vi "TPM with correction version 10-3-compare-1 scale factor_descan_20191023_WF.vi"() -> ()   [LabVIEW 2018]
uses:
  Casao LabVIEW SDK 1.0.5/Haso/Data Haso/Wavefront parameters.ctl
  Casao LabVIEW SDK 1.0.5/Casao/Casao/Loop prefs.ctl
  Casao LabVIEW SDK 1.0.5/Haso/Data Haso/DataHaso.ctl
  <vilib>/Utility/file.llb/Read From Spreadsheet File (DBL).vi
  <vilib>/Utility/file.llb/Write To Spreadsheet File (DBL).vi
panel:
  in  "galvo scan?":bool
  out "error out 1":errorcluster={"status"=FALSE, "code"=25, "source"=""}
  out "error out 3":errorcluster={"status"=FALSE, "code"=25, "source"=""}
  out "error out 2":errorcluster={"status"=FALSE, "code"=25, "source"=""}
  out "error out 0":errorcluster={"status"=FALSE, "code"=25, "source"=""}
  in  "Descan  Rescan":bool
  in  "Camera              WF sensor":bool
  in  "Scale factor":dbl=1.0
  out "output path":path
  out "Model Coefficients (µm) after":sgl[](array[numeric])
  out "Model Coefficients (µm) before":sgl[](array[numeric])
  in  "stop":bool
  out "Slice now":dbl
  in  "Iteration #":u16(ring)=1 items=["1"=1, "2"=2, "3"=3, "4"=4, "5"=5]
  in  "AoExp Time":dbl(ring)=0.5 items=["0.2s"=0.2, "0.5s"=0.5, "1.0s"=1.0, "1.5s"=1.5]
  out "after correction":T1
  in  "Filter y tilt":bool=TRUE
  in  "Filter x tilt":bool=TRUE
  in  "Curvature filter":bool=TRUE
  out "PV":dbl
  out "RMS":dbl
  in  "Matrix path":path=path "C:/Users/user/Desktop/YD/20191025/CM.aomc"
  in  "Offset path":path=path "D:/SystemAlignment/syste_aberration_20191015.dat"
  out "Camera image":u32[][](graph)
  out "RMS":dbl
  out "PV":dbl
  out "before correction":T1
  in  "Curvature filter":bool=TRUE
  in  "Filter y tilt":bool=TRUE
  in  "Filter x tilt":bool=TRUE
  out "after correction":dbl[][](graph) caption="Wavefront"
  out "before correction":dbl[][](graph) caption="Wavefront"
  in  "ImExp Time (s)":dbl(ring)=0.5 items=["0.2"=0.2, "0.5"=0.5, "1.0"=1.0, "4.0"=4.0, "8.0"=8.0]
  in  "Step size(um)":dbl
  in  "Laser Power%(0-100)":dbl=50.0
  in  "Slices #":dbl=1.0
  in  "Average Frame #":dbl=5.0
  in  "Correction":bool
  # "OFF"
  # "ON"
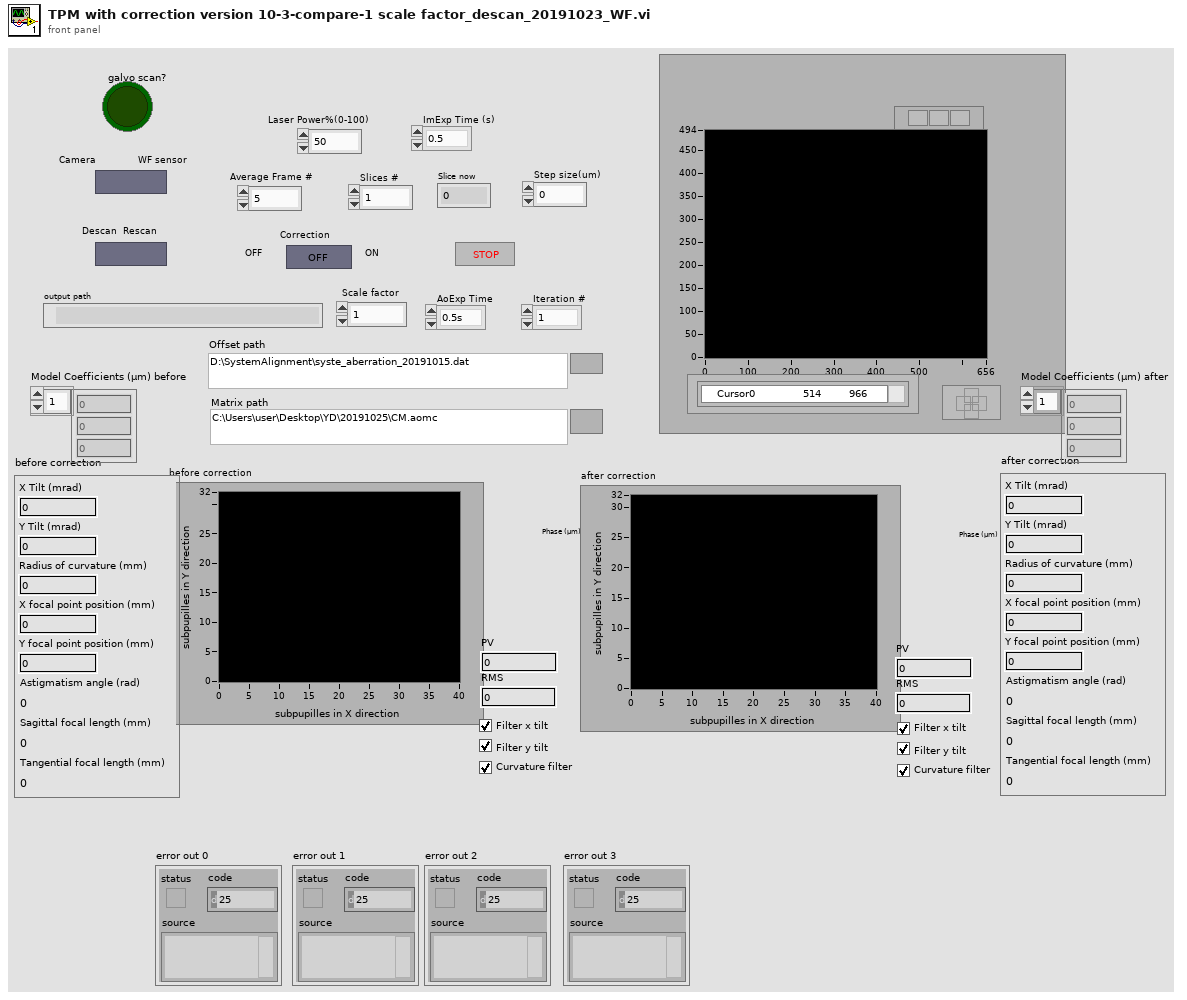
[diagram p1: front panel]
types:
  T1 = typedef "Wavefront parameters.ctl" = cluster{"X Tilt (mrad)":sgl, "Y Tilt (mrad)":sgl, "Radius of curvature (mm)":sgl, "X focal point position (mm)":sgl, "Y focal point position (mm)":sgl, "Astigmatism angle (rad)":sgl, "Sagittal focal length (mm)":sgl, "Tangential focal length (mm)":sgl}
  T2 = typedef "Loop prefs.ctl" = cluster{"Filter tilt on measurement (closed loop)":bool, "Correction gain (closed loop)":sgl, "Limit of subapertures off in CGP (%)":sgl, "Limit of saturated actuators (%)":sgl}
  T3 = cluster{"Filtre tilt X":bool, "Filtre tilt Y":bool, "Filtre courbure":bool}
  T4 = typedef "DataHaso.ctl" = i32
  T5 = cluster{"Measurement":T4, "Target":T4, "Manual target":T4}
  T6 = cluster{"Target for tilt":T4, "Target for focus":T4, "Target for all other aberrations":T4}
  T7 = typedef "Camera.ctl" = i32
  T8 = typedef "PhaseModul.ctl" = i32
  T9 = typedef "Haso.ctl" = i32
  T10 = typedef "Casao.ctl" = i32
  T11 = typedef "Image Compat.ctl" = cluster{"Signed/unsigned":bool, "Number of bits":T12, "Internal object id":i32, "Internal data id":i32}
  T12 = typedef "Data alignment enum.ctl" = enum16{"8", "16", "32"}
  T13 = typedef "Reconstruction prefs.ctl" = cluster{"Reconstruction type":enum16{"Modal", "Zonal"}, "Polynomial type":enum16{"Zernike", "Legendre"}, "Modal reconstruction prefs":T14, "Zonal reconstruction prefs":T17}
  T14 = typedef "Modal reconstruction prefs.ctl" = cluster{"Number of coefficients":u32, "Filtered coefficients":u32[], "RMS Zernike normalization":bool, "Matrix inversion method":u16, "Add zonal residual to modal fit ":bool, "Detection prefs":T15}
  T15 = typedef "PupilDetectionPrefs.ctl" = cluster{"Automatic pupil detection":bool, "Central occultation pupil":bool, "Semi-automatic pupil detection (find radius)":bool, "Semi-automatic pupil detection (find center)":bool, "Automatic pupil detection mode":enum16{"Contained", "Containing"}, "Start coordinates":cluster{"Pupil center (Zernike)":T16, "Pupil radius (Zernike)":sgl, "Pupil center (Legendre)":T16, "Pupil halfsize (Legendre)":T16}}
  T16 = typedef "Point2Df.ctl" = cluster{"X":sgl, "Y":sgl}
  T17 = typedef "Zonal reconstruction prefs.ctl" = cluster{"Number of weak iterations":u16, "Number of max iterations":u32, "Residual limit":sgl}
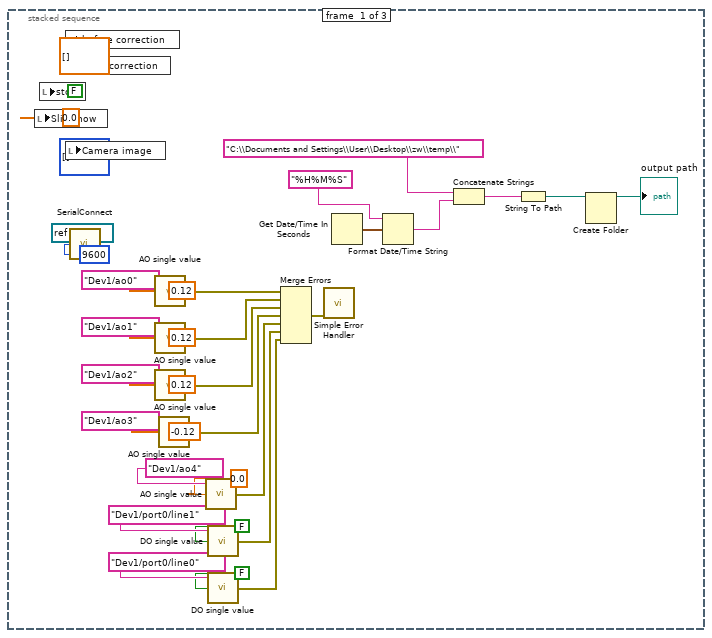
[diagram p2: hidden frame]
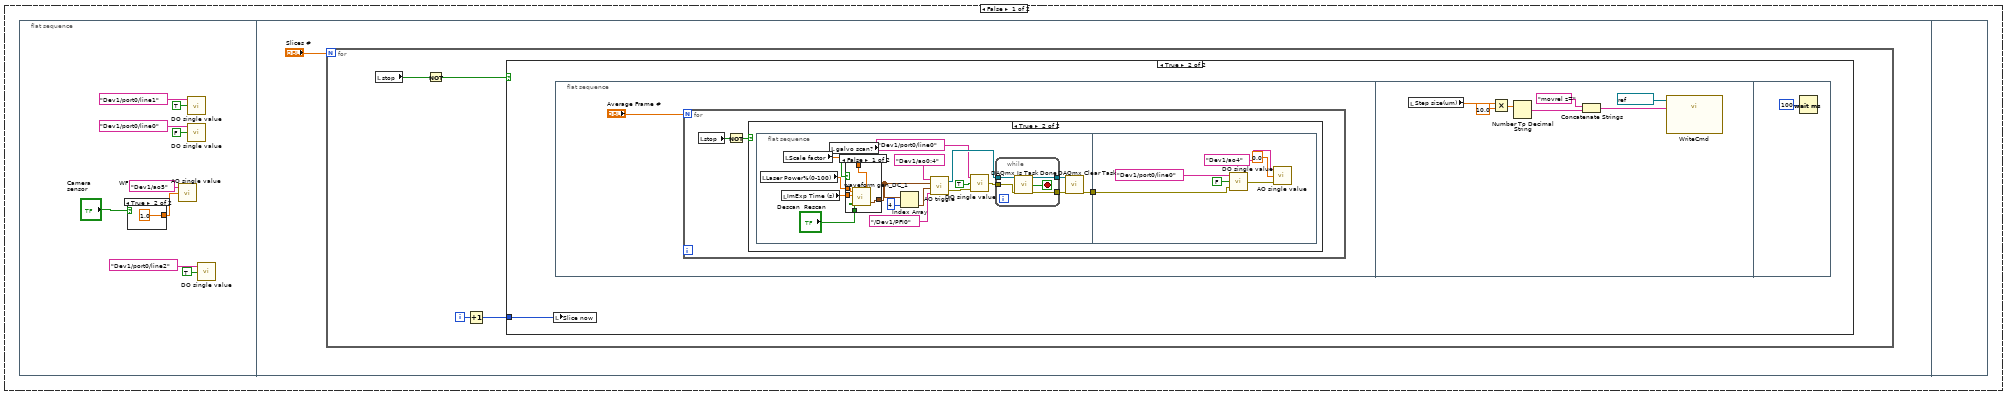
[diagram p3: hidden frame]
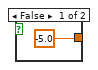
[diagram p4: hidden frame]
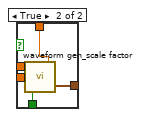
[diagram p7: hidden frame]
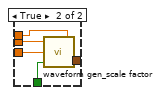
[diagram p10: hidden frame]
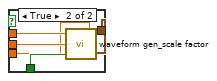
[diagram p11: hidden frame]
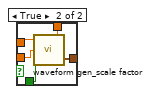
[diagram p12: hidden frame]
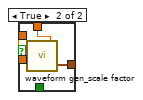
[diagram p16: hidden frame]
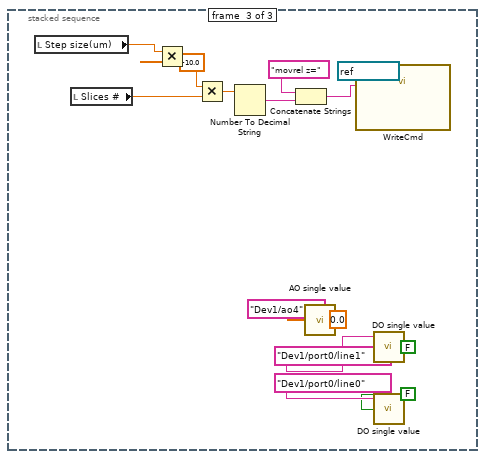
[diagram p17: hidden frame]
diagram:
  # "ao0: stim G A \nao1: stim G B\nao2: Emission G A\nao3: Emission G B\nao4: Pockel Cell\nao5: Emission steering G\nao6: stage z piezo\nPFI0: andor send out trigger\nP0.0: andor send in trigger?"
  n1 = stacked-sequence {
    tunnel: "galvo scan?" -> [_ w37 _]
    frame #0 {
      w35 = dbl[][] [] ("before correction")
      n2 = local write "Slice now"(0.0 ("Slice now")) -> ()
      n3 = local write "stop"(FALSE ("stop")) -> ()
      n4 = local write "before correction"(w35) -> ()
      n5 = local write "Camera image"(u32[][] [] ("Camera image")) -> ()
      n6 = local write "after correction"(w35) -> ()
      n7 = call "SerialConnect.vi"("baud rate (9600)"=u32 9600, "VISA resource name"=refnum<visa-resource-name> "COM1") -> ()  [unwired: 1 in, 3 out]
      n8 = call "AO single value.vi"("data"=0.12, "physical channels"=tag "Dev1/ao0") -> ("error out"=w18:errorcluster)  [unwired: 1 in]
      n9 = call "AO single value.vi"("data"=0.12, "physical channels"=tag "Dev1/ao1") -> ("error out"=w17:errorcluster)  [unwired: 1 in]
      n10 = call "AO single value.vi"("data"=0.12, "physical channels"=tag "Dev1/ao2") -> ("error out"=w16:errorcluster)  [unwired: 1 in]
      n11 = call "AO single value.vi"("data"=-0.12, "physical channels"=tag "Dev1/ao3") -> ("error out"=w15:errorcluster)  [unwired: 1 in]
      n12 = call "AO single value.vi"("data"=0.0, "physical channels"=tag "Dev1/ao4") -> ("error out"=w14:errorcluster)  [unwired: 1 in]
      n13 = call "DO single value.vi"("data"=FALSE, "lines"=tag "Dev1/port0/line1") -> ("error out"=w13:errorcluster)  [unwired: 1 in]
      n14 = call "DO single value.vi"("data"=FALSE, "lines"=tag "Dev1/port0/line0") -> ("error out"=w11:errorcluster)  [unwired: 1 in]
      n15 = Merge Errors(w18, w17, w16, w15, w14, w13, w11) -> (w12:errorcluster)
      n16 = call <vilib>:"Simple Error Handler.vi"("error in (no error)"=w12) -> ()  [unwired: 4 in, 5 out]
      n17 = Get Date/Time In Seconds() -> (seconds since 1Jan1904=w8:timestamp)
      n18 = Format Date/Time String(time format string (%c)="%H%M%S", seconds (now)=w8) -> (date/time string=w5:string)  [unwired: 1 in]
      n19 = Concatenate Strings("C:\\Documents and Settings\\User\\Desktop\\zw\\temp\\" ("string"), w5) -> (w4:string)
      n20 = String To Path(string=w4) -> (path=w3:path)
      n21 = Create Folder(path (use dialog)=w3) -> (created path=→"output path":path)  [unwired: 2 in, 2 out]
    }
    frame #1 {
      n22 = case shown="True" "Correction" {
        tunnel: w37 -> [_ w107]
        frame False {
          n23 = flat-sequence {
            frame #0 {
              n24 = case shown="True" "Camera              WF sensor" {
                tunnel: [-5.0 ("data") 1.0 ("data")] -> w42
                frame False {
                }
                frame True {
                }
              }
              n25 = call "AO single value.vi"("data"=w42, "physical channels"=tag "Dev1/ao5") -> ()  [unwired: 1 in, 1 out]
              n26 = call "DO single value.vi"("data"=TRUE, "lines"=tag "Dev1/port0/line1") -> ()  [unwired: 1 in, 1 out]
              n27 = call "DO single value.vi"("data"=FALSE, "lines"=tag "Dev1/port0/line0") -> ()  [unwired: 1 in, 1 out]
              n28 = call "DO single value.vi"("data"=TRUE, "lines"=tag "Dev1/port0/line2") -> ()  [unwired: 1 in, 1 out]
            }
            frame #1 {
              n29 = for {
                N: "Slices #" -> [_]
                i -> [w54]
                n30 = local read "stop"() -> (w52:bool)
                n31 = Not(x=w52) -> (.not. x?=w51:bool)
                n32 = Increment(x=w54) -> (x+1=w53:i32)
                n33 = case shown="True" w51 {
                  tunnel: w53 -> [_ w55]
                  frame False {
                  }
                  frame True {
                    n34 = local write "Slice now"(w55) -> ()
                    n35 = flat-sequence {
                      frame #0 {
                        n36 = for {
                          N: "Average Frame #" -> [_]
                          n37 = local read "stop"() -> (w57:bool)
                          n38 = Not(x=w57) -> (.not. x?=w58:bool)
                          n39 = case shown="True" w58 {
                            frame False {
                            }
                            frame True {
                              n40 = flat-sequence {
                                tunnel: [w66] -> w59
                                tunnel: w59 -> [w94]
                                frame #0 {
                                n41 = local read "Laser Power%(0-100)"() -> (w63:dbl)
                                n42 = local read "ImExp Time (s)"() -> (w64:dbl)
                                n43 = local read "Scale factor"() -> (w62:dbl)
                                n44 = local read "galvo scan?"() -> (w60:bool)
                                n45 = case shown="False" w60 {
                                tunnel: [w82 w87] -> w65
                                tunnel: w64 -> [w79 w86]
                                tunnel: w63 -> [w80 w85]
                                tunnel: w62 -> [w81 w84]
                                tunnel: "Descan  Rescan" -> [w78 w83]
                                frame False {
                                n46 = call "waveform gen_DC_1.vi"("Scale factor"=w81, "Boolean"=w78, "Exposure Time (s)"=w79, "Laser Power%(0-100)"=w80) -> ("waveform"=w82:waveform(dbl)[])
                                }
                                frame True {
                                n47 = call "waveform gen_scale factor.vi"("Scale factor"=w84, "Boolean"=w83, "Exposure Time (s)"=w86, "Laser Power%(0-100)"=w85) -> ("waveform"=w87:waveform(dbl)[])
                                }
                                }
                                n48 = Index Array(array=w65, index=4) -> (element=w74:waveform(dbl))
                                n49 = call "AO triggle.vi"("physical channels"=tag "Dev1/ao0:4", "data"=w65, "waveform"=w74, "trig source"=tag "/Dev1/PFI0") -> ("task out"=w71:refnum<k21>, "error out"=w68:errorcluster)  [unwired: 1 in]
                                n50 = call "DO single value.vi"("error in"=w68, "data"=TRUE, "lines"=tag "Dev1/port0/line0") -> ("error out"=w67:errorcluster)
                                n51 = while {
                                tunnel: [w92] -> w77
                                tunnel: [w91] -> w76
                                tunnel: w71 -> [w89]
                                tunnel: w67 -> [w88]
                                stop <- w90 stop-if-true
                                n52 = call <vilib>:"DAQmx Is Task Done.vi"("task/channels in"=w89, "error in"=w88) -> ("task out"=w92:refnum<k21>, "task done?"=w90:bool, "error out"=w91:errorcluster)  [unwired: 11 in]
                                }
                                n53 = call <vilib>:"DAQmx Clear Task.vi"("task in"=w77, "error in"=w76) -> ("error out"=w66:errorcluster)  [unwired: 13 in]
                                }
                                frame #1 {
                                n54 = call "DO single value.vi"("error in"=w94, "data"=FALSE, "lines"=tag "Dev1/port0/line0") -> ("error out"=w93:errorcluster)
                                n55 = call "AO single value.vi"("error in"=w93, "data"=0.0, "physical channels"=tag "Dev1/ao4") -> ()  [unwired: 1 out]
                                }
                              }
                            }
                          }
                        }
                      }
                      frame #1 {
                        n56 = local read "Step size(um)"() -> (w99:dbl)
                        n57 = Multiply(x=w99, y=10.0) -> (x*y=w101:dbl)
                        n58 = Number To Decimal String(number=w101) -> (decimal integer string=w104:string)  [unwired: 1 in]
                        n59 = Concatenate Strings("movrel z=", w104) -> (w103:string)
                        n60 = call "WriteCmd.vi"("Command"=w103, "VISA resource name"=refnum<visa-resource-name> "COM1") -> ()  [unwired: 1 in, 1 out]
                      }
                      frame #2 {
                        n61 = Wait (ms)(milliseconds to wait=u32 100) -> ()  [unwired: 1 out]
                      }
                    }
                  }
                }
              }
            }
            frame #2 {
            }
          }
        }
        frame True {
          n62 = flat-sequence {
            tunnel: [w116] -> w115
            tunnel: [w125] -> w114
            tunnel: [w124] -> w113
            tunnel: [w116] -> w112
            tunnel: [w123] -> w111
            tunnel: [w122] -> w109
            tunnel: [w117] -> w108
            tunnel: w115 -> [w143]
            tunnel: w114 -> [w142]
            tunnel: w113 -> [w141]
            tunnel: w112 -> [w137]
            tunnel: w111 -> [w135]
            tunnel: [w140] -> w110
            tunnel: w109 -> [w139]
            tunnel: w108 -> [w133]
            tunnel: w107 -> [w132]
            tunnel: w110 -> [w718]
            frame #0 {
              n63 = call "AO single value.vi"("data"=0.0, "physical channels"=tag "Dev1/ao4") -> ()  [unwired: 1 in, 1 out]
              n64 = local read "AoExp Time"() -> (w126:dbl)
              n65 = call-poly <vilib>:"Read From Spreadsheet File.vi"("format (%.3f)"="%.8f", "file path (dialog if empty)"="Offset path") -> ("first row"=w117:dbl[])  [unwired: 5 in, 4 out]
              n66 = call "DO single value.vi"("data"=TRUE, "lines"=tag "Dev1/port0/line1") -> ()  [unwired: 1 in, 1 out]
              n67 = call "DO single value.vi"("data"=FALSE, "lines"=tag "Dev1/port0/line0") -> ()  [unwired: 1 in, 1 out]
              n68 = call "AO init.vi"("Exposure duration specified (s)"=w126, "Commands in"=w117, "Matrix path"="Matrix path") -> ("error out"=w116:errorcluster, "Camera"=w125:T7, "Mirror"=w122:T8, "Haso"=w124:T9, "Casao"=w123:T10)  [unwired: 3 in, 1 out]
              "error out 0" <- w116
            }
            frame #1 {
              n69 = local read "Slices #"() -> (w144:dbl)
              n70 = call "Casao Set Preferences.vi"("error in (no error)"=w137, "Loop preferences"=T2 {"Filter tilt on measurement (closed loop)"=FALSE, "Correction gain (closed loop)"=0.75, "Limit of subapertures off in CGP (%)"=0.0, "Limit of saturated actuators (%)"=0.0}, "Casao"=w135) -> ("error out"=w136:errorcluster, "Casao (dup)"=w134:T10)  [unwired: 3 in]
              n71 = for {
                N: w144 -> [_]
                tunnel: w143 -> [w161]
                tunnel: w142 -> [w160]
                tunnel: w141 -> [w159]
                tunnel: w136 -> [w147]
                tunnel: [w158] -> w140
                tunnel: w139 -> [w149]
                tunnel: w134 -> [w157]
                tunnel: w133 -> [w150]
                tunnel: w132 -> [w145]
                i -> [w153]
                n72 = local read "stop"() -> (w155:bool)
                n73 = call "PhaseModul apply command.vi"("error in (no error)"=w147, "Commands in"=w150, "Mirror"=w149) -> ("error out"=w146:errorcluster, "Mirror (dup)"=w148:T8)  [unwired: 2 in, 1 out]
                n74 = Increment(x=w153) -> (x+1=w156:i32)
                n75 = local write "Slice now"(w156) -> ()
                n76 = Not(x=w155) -> (.not. x?=w154:bool)
                n77 = case shown="True" w154 {
                  tunnel: w161 -> [_ w197]
                  tunnel: w160 -> [_ w196]
                  tunnel: w159 -> [_ w195]
                  tunnel: w146 -> [_ w194]
                  tunnel: [w162 w191] -> w158
                  tunnel: w148 -> [_ w193]
                  tunnel: w157 -> [w162 w192]
                  tunnel: w145 -> [_ w163]
                  frame False {
                  }
                  frame True {
                    n78 = flat-sequence {
                      tunnel: w192 -> [w203]
                      tunnel: w193 -> [w204]
                      tunnel: w194 -> [w205]
                      tunnel: w195 -> [w206]
                      tunnel: w196 -> [w207]
                      tunnel: w197 -> [w208]
                      tunnel: [w208] -> w169
                      tunnel: [w207] -> w168
                      tunnel: [w206] -> w167
                      tunnel: [w205] -> w166
                      tunnel: [w204] -> w165
                      tunnel: [w203] -> w164
                      tunnel: w163 -> [w198]
                      tunnel: [w257] -> w190
                      tunnel: [w256] -> w189
                      tunnel: [w255] -> w188
                      tunnel: [w250] -> w187
                      tunnel: [w251] -> w186
                      tunnel: [w252] -> w185
                      tunnel: w169 -> [w257]
                      tunnel: w168 -> [w256]
                      tunnel: w167 -> [w255]
                      tunnel: w166 -> [w251]
                      tunnel: w165 -> [w252]
                      tunnel: w164 -> [w250]
                      tunnel: w190 -> [w299]
                      tunnel: w189 -> [w298]
                      tunnel: w188 -> [w297]
                      tunnel: w187 -> [w296]
                      tunnel: w186 -> [w295]
                      tunnel: [w275] -> w184
                      tunnel: [w274] -> w183
                      tunnel: [w270] -> w182
                      tunnel: [w268] -> w181
                      tunnel: [w266] -> w180
                      tunnel: w185 -> [w261]
                      tunnel: [w260] -> w179
                      tunnel: [w258] -> w178
                      tunnel: w184 -> [w452]
                      tunnel: w183 -> [w451]
                      tunnel: w182 -> [w449]
                      tunnel: w181 -> [w448]
                      tunnel: w180 -> [w447]
                      tunnel: [w446] -> w177
                      tunnel: w179 -> [w445]
                      tunnel: [w444] -> w176
                      tunnel: [w443] -> w175
                      tunnel: [w442] -> w174
                      tunnel: [w441] -> w173
                      tunnel: [w440] -> w172
                      tunnel: w178 -> [w439]
                      tunnel: [w439] -> w171
                      tunnel: w177 -> [w670]
                      tunnel: [w670] -> w170
                      tunnel: w176 -> [w660]
                      tunnel: w175 -> [w659]
                      tunnel: w174 -> [w658]
                      tunnel: w173 -> [w648]
                      tunnel: w172 -> [w649]
                      tunnel: w171 -> [w647]
                      tunnel: w170 -> [w671]
                      tunnel: [w671] -> w191
                      frame #0 {
                        n79 = local read "Average Frame #"() -> (w202:dbl)
                        n80 = Wait (ms)(milliseconds to wait=u32 100) -> ()  [unwired: 1 out]
                        n81 = call "AO single value.vi"("data"=-5.0, "physical channels"=tag "Dev1/ao5") -> ()  [unwired: 1 in, 1 out]
                        n82 = for {
                          N: w202 -> [_]
                          tunnel: w198 -> [w209]
                          n83 = local read "stop"() -> (w210:bool)
                          n84 = Not(x=w210) -> (.not. x?=w211:bool)
                          n85 = case shown="True" w211 {
                            tunnel: w209 -> [_ w212]
                            frame False {
                            }
                            frame True {
                              n86 = flat-sequence {
                                tunnel: w212 -> [w213]
                                frame #0 {
                                n87 = local read "Laser Power%(0-100)"() -> (w215:dbl)
                                n88 = local read "ImExp Time (s)"() -> (w216:dbl)
                                n89 = local read "Scale factor"() -> (w214:dbl)
                                n90 = case shown="False" w213 {
                                tunnel: [w231 w239] -> w218
                                tunnel: TRUE ("Boolean") -> [w230 w238]
                                tunnel: w216 -> [w232 w237]
                                tunnel: w215 -> [w233 w236]
                                tunnel: w214 -> [w234 w235]
                                frame False {
                                n91 = call "waveform gen_DC_1.vi"("Scale factor"=w234, "Boolean"=w230, "Exposure Time (s)"=w232, "Laser Power%(0-100)"=w233) -> ("waveform"=w231:waveform(dbl)[])
                                }
                                frame True {
                                n92 = call "waveform gen_scale factor.vi"("Scale factor"=w235, "Boolean"=w238, "Exposure Time (s)"=w237, "Laser Power%(0-100)"=w236) -> ("waveform"=w239:waveform(dbl)[])
                                }
                                }
                                n93 = Index Array(array=w218, index=4) -> (element=w226:waveform(dbl))
                                n94 = call "AO triggle.vi"("physical channels"=tag "Dev1/ao0:4", "data"=w218, "waveform"=w226, "trig source"=tag "/Dev1/PFI0") -> ("task out"=w223:refnum<k21>, "error out"=w220:errorcluster)  [unwired: 1 in]
                                n95 = call "DO single value.vi"("error in"=w220, "data"=TRUE, "lines"=tag "Dev1/port0/line0") -> ("error out"=w219:errorcluster)
                                n96 = while {
                                tunnel: [w244] -> w229
                                tunnel: [w243] -> w228
                                tunnel: w223 -> [w241]
                                tunnel: w219 -> [w240]
                                stop <- w242 stop-if-true
                                n97 = call <vilib>:"DAQmx Is Task Done.vi"("task/channels in"=w241, "error in"=w240) -> ("task out"=w244:refnum<k21>, "task done?"=w242:bool, "error out"=w243:errorcluster)  [unwired: 11 in]
                                }
                                n98 = call <vilib>:"DAQmx Clear Task.vi"("task in"=w229, "error in"=w228) -> ()  [unwired: 13 in, 1 out]
                                }
                                frame #1 {
                                n99 = call "AO single value.vi"("data"=0.0, "physical channels"=tag "Dev1/ao4") -> ()  [unwired: 1 in, 1 out]
                                n100 = call "DO single value.vi"("data"=FALSE, "lines"=tag "Dev1/port0/line0") -> ()  [unwired: 1 in, 1 out]
                                }
                              }
                            }
                          }
                        }
                      }
                      frame #1 {
                        n101 = call "AO single value.vi"("data"=1.0, "physical channels"=tag "Dev1/ao5") -> ("error out"=→"error out 1":errorcluster)  [unwired: 1 in]
                      }
                      frame #2 {
                        n102 = flat-sequence {
                          tunnel: [w309] -> w294
                          tunnel: [w308] -> w293
                          tunnel: [w307] -> w292
                          tunnel: [w306] -> w291
                          tunnel: [w305] -> w290
                          tunnel: w297 -> [w307]
                          tunnel: w298 -> [w308]
                          tunnel: w299 -> [w309]
                          tunnel: [w304] -> w289
                          tunnel: w296 -> [w304]
                          tunnel: [w303] -> w288
                          tunnel: w295 -> [w303]
                          tunnel: [w302] -> w262
                          tunnel: w261 -> [w302]
                          tunnel: w294 -> [w335]
                          tunnel: w293 -> [w336]
                          tunnel: w292 -> [w337]
                          tunnel: [w337] -> w287
                          tunnel: [w334] -> w286
                          tunnel: [w328] -> w285
                          tunnel: [w333] -> w284
                          tunnel: w291 -> [w333]
                          tunnel: [w332] -> w283
                          tunnel: w290 -> [w332]
                          tunnel: [w331] -> w282
                          tunnel: w289 -> [w331]
                          tunnel: [w330] -> w281
                          tunnel: w288 -> [w330]
                          tunnel: [w329] -> w263
                          tunnel: w262 -> [w329]
                          tunnel: w287 -> [w349]
                          tunnel: [w349] -> w278
                          tunnel: [w348] -> w279
                          tunnel: w286 -> [w348]
                          tunnel: [w347] -> w280
                          tunnel: w285 -> [w347]
                          tunnel: w284 -> [w342]
                          tunnel: w283 -> [w341]
                          tunnel: [w340] -> w277
                          tunnel: w282 -> [w340]
                          tunnel: [w339] -> w276
                          tunnel: w281 -> [w339]
                          tunnel: [w338] -> w264
                          tunnel: w263 -> [w338]
                          tunnel: w280 -> [w431]
                          tunnel: w279 -> [w392]
                          tunnel: w278 -> [w393]
                          tunnel: w277 -> [w417]
                          tunnel: w276 -> [w416]
                          tunnel: [w396] -> w273
                          tunnel: [w395] -> w272
                          tunnel: [w394] -> w271
                          tunnel: [w393] -> w269
                          tunnel: [w392] -> w267
                          tunnel: [w391] -> w265
                          tunnel: w264 -> [w390]
                          tunnel: [w390] -> w259
                          tunnel: [w364] -> w258
                          tunnel: [w437] -> w274
                          tunnel: [w438] -> w275
                          tunnel: w273 -> [w438]
                          tunnel: w272 -> [w437]
                          tunnel: w271 -> [w436]
                          tunnel: [w435] -> w270
                          tunnel: w269 -> [w435]
                          tunnel: [w434] -> w268
                          tunnel: w267 -> [w434]
                          tunnel: [w433] -> w266
                          tunnel: w265 -> [w433]
                          tunnel: [w432] -> w260
                          tunnel: w259 -> [w432]
                          frame #0 {
                            n103 = local read "Laser Power%(0-100)"() -> (w315:dbl)
                            n104 = local read "AoExp Time"() -> (w314:dbl)
                            n105 = local read "Scale factor"() -> (w301:dbl)
                            n106 = local read "galvo scan?"() -> (w300:bool)
                            n107 = case shown="False" w300 {
                              tunnel: FALSE ("Boolean") -> [w322 w327]
                              tunnel: w315 -> [w320 w326]
                              tunnel: w314 -> [w319 w325]
                              tunnel: [w318 w324] -> w313
                              tunnel: w301 -> [w321 w323]
                              frame False {
                                n108 = call "waveform gen_DC_1.vi"("Scale factor"=w321, "Boolean"=w322, "Exposure Time (s)"=w319, "Laser Power%(0-100)"=w320) -> ("waveform"=w318:waveform(dbl)[])
                              }
                              frame True {
                                n109 = call "waveform gen_scale factor.vi"("Scale factor"=w323, "Boolean"=w327, "Exposure Time (s)"=w325, "Laser Power%(0-100)"=w326) -> ("waveform"=w324:waveform(dbl)[])
                              }
                            }
                            n110 = Index Array(array=w313, index=4) -> (element=w312:waveform(dbl))
                            n111 = call "AO triggle.vi"("physical channels"=tag "Dev1/ao0:4", "data"=w313, "waveform"=w312, "trig source"=tag "/Dev1/PFI0") -> ("task out"=w306:refnum<k21>, "error out"=w305:errorcluster)  [unwired: 1 in]
                          }
                          frame #1 {
                            n112 = call "Camera Start.vi"("error in (no error)"=w335, "camera"=w336) -> ("error out"=w328:errorcluster, "camera (dup)"=w334:T7)  [unwired: 4 in]
                            "error out 2" <- w328
                          }
                          frame #2 {
                            n113 = while {
                              tunnel: [w354] -> w344
                              tunnel: [w353] -> w343
                              tunnel: w342 -> [w351]
                              tunnel: w341 -> [w350]
                              stop <- w352 stop-if-true
                              n114 = call <vilib>:"DAQmx Is Task Done.vi"("task/channels in"=w351, "error in"=w350) -> ("task out"=w354:refnum<k21>, "task done?"=w352:bool, "error out"=w353:errorcluster)  [unwired: 11 in]
                            }
                            n115 = call "DO single value.vi"("data"=TRUE, "lines"=tag "Dev1/port0/line0") -> ()  [unwired: 1 in, 1 out]
                            n116 = call <vilib>:"DAQmx Clear Task.vi"("task in"=w344, "error in"=w343) -> ()  [unwired: 13 in, 1 out]
                          }
                          frame #3 {
                            n117 = call "Camera Get image.vi"("error in (no error)"=w431, "camera"=w392) -> ("error out"=w413:errorcluster, "Image"=w414:T11, "camera (dup)"=w415:T7)  [unwired: 3 in]
                            n118 = call "Camera Stop.vi"("error in (no error)"=w413, "camera"=w415) -> ()  [unwired: 4 in, 2 out]
                            n119 = call "Image get data.vi"("error in (no error)"=w413, "Image Compat"=w414) -> ("error out"=w355:errorcluster, "Array"=w412:u32[][], "Image Compat (dup)"=w403:T11)  [unwired: 3 in]
                            "error out 3" <- w355
                            n120 = call "AO single value.vi"("data"=0.0, "physical channels"=tag "Dev1/ao4") -> ()  [unwired: 1 in, 1 out]
                            n121 = local write "Camera image"(w412) -> ()
                            n122 = call "Haso compute slopes.vi"("error in (no error)"=w355, "Image Compat"=w403, "Haso"=w393) -> ("error out"=w362:errorcluster, "Data Haso"=w366:T4)  [unwired: 1 in, 2 out]
                            n123 = call "DO single value.vi"("data"=FALSE, "lines"=tag "Dev1/port0/line0") -> ()  [unwired: 1 in, 1 out]
                            n124 = call "DataHaso ctor copie.vi"("error in (no error)"=w362, "DataHaso"=w366) -> ("error out"=w361:errorcluster, "new DataHaso"=w364:T4, "DataHaso (dup)"=w363:T4)  [unwired: 3 in]
                            n125 = call "DataHaso get reconstruction prefs.vi"("error in (no error)"=w361, "Data Haso"=w363) -> ("error out"=w377:errorcluster, "Reconstruction Preferences"=w373:T13, "Data Haso (dup)"=w376:T4)  [unwired: 3 in]
                            n126 = Bundle By Name(cluster=w373, "Reconstruction type"=enum16{"Modal", "Zonal"}."Modal", "Polynomial type"=enum16{"Zernike", "Legendre"}."Zernike", "Modal reconstruction prefs.Number of coefficients"=u32 32) -> (w372:T13)
                            n127 = call "DataHaso set reconstruction prefs.vi"("error in (no error)"=w377, "Reconstruction Preferences"=w372, "Data Haso"=w376) -> ("error out"=w374:errorcluster, "Data Haso (dup)"=w375:T4)  [unwired: 3 in]
                            n128 = call "DataHaso get modal coefficients.vi"("error in (no error)"=w374, "Data Haso"=w375) -> ("error out"=w367:errorcluster, "Coefficients (µm)"=w378:sgl[], "Data Haso (dup)"=w368:T4)  [unwired: 3 in]
                            "Model Coefficients (µm) before" <- w378
                            n129 = Bundle By Name(cluster=T3 {"Filtre tilt X"=FALSE, "Filtre tilt Y"=FALSE, "Filtre courbure"=FALSE} ("Filtre"), "Filtre tilt X"="Filter x tilt", "Filtre tilt Y"="Filter y tilt", "Filtre courbure"="Curvature filter") -> (w398:T3)
                            n130 = call "DataHaso parameters.vi"("error in (no error)"=w367, "Data Haso"=w368) -> ("error out"=w410:errorcluster, "Parameters"=w386:T1, "Data Haso (dup)"=w411:T4)  [unwired: 3 in]
                            "before correction" <- w386
                            n131 = control-ref of="before correction"() -> (w397:refnum<vi>)
                            n132 = Cluster To Array(cluster=w386) -> (array=w387:sgl[])
                            n133 = call "DataHaso filter tilt or curvature.vi"("error in (no error)"=w410, "Filter (default: all true)"=w398, "Data Haso"=w411) -> ("error out"=w408:errorcluster, "Data Haso (dup)"=w409:T4)  [unwired: 3 in]
                            n134 = local read "Slice now"() -> (w380:dbl)
                            n135 = call "DataHaso phase.vi"("error in (no error)"=w408, "Data Haso"=w409) -> ("error out"=w406:errorcluster, "Phase (µm)"=w407:i32, "Data Haso (dup)"=w365:T4)  [unwired: 3 in]
                            n136 = Number To Decimal String(number=w380) -> (decimal integer string=w382:string)  [unwired: 1 in]
                            n137 = call "Formatter Intensity Graph.vi"("error in (no error)"=w406, "Intensity Graph"=w397, "Surface with pupil"=w407) -> ("error out"=w404:errorcluster, "Surface with pupil (dup)"=w405:i32)  [unwired: 2 in, 1 out]
                            n138 = call "Surface with pupil get stats.vi"("error in (no error)"=w404, "Surface Avec Pupille"=w405) -> ("error out"=w391:errorcluster, "PV"=w389:sgl, "RMS"=w388:dbl)  [unwired: 2 in, 1 out]
                            "PV" <- w389
                            "RMS" <- w388
                            n139 = local read "output path"() -> (w358:path)
                            n140 = Concatenate Strings("before_slice", w382, ".dat") -> (w357:string)
                            n141 = Build Path(base path=w358, name or relative path=w357) -> (appended path=w356:path)
                            n142 = Build Array (concatenate)(w389, w388, w387, w378) -> (w385:dbl[])
                            n143 = Merge Errors(w391, w416) -> (w426:errorcluster)
                            n144 = Bundle By Name(cluster=T6 {"Target for tilt"=0, "Target for focus"=0, "Target for all other aberrations"=0} ("References"), "Target for tilt"=w364, "Target for focus"=w364) -> (w429:T6)
                            n145 = call "DataHaso ctor copie.vi"("error in (no error)"=w426, "DataHaso"=w365) -> ("error out"=w428:errorcluster, "new DataHaso"=w427:T4)  [unwired: 3 in, 1 out]
                            n146 = call-poly <vilib>:"Write To Spreadsheet File.vi"("transpose? (no:F)"=TRUE, "format (%.3f)"="%.6f", "1D data"=w385, "file path (dialog if empty)"=w356) -> ()  [unwired: 4 in, 1 out]
                            n147 = call "Casao Compute target.vi"("error in (no error)"=w428, "Targets"=w429, "DataHaso"=w427, "Casao"=w417) -> ("error out"=w424:errorcluster, "DataHaso (dup)"=w394:T4, "Casao (dup)"=w425:T10)  [unwired: 1 out]
                            n148 = Bundle By Name(cluster=T5 {"Measurement"=0, "Target"=0, "Manual target"=0} ("Slopes"), "Measurement"=w365, "Target"=w394) -> (w423:T5)
                            n149 = call "Casao get correction commands.vi"("Casao"=w425, "Slopes"=w423, "error in (no error)"=w424) -> ("Casao (dup)"=w396:T10, "Commands"=w420:sgl[], "error out"=w421:errorcluster)  [unwired: 2 in, 2 out]
                            n150 = call "PhaseModul apply command.vi"("error in (no error)"=w421, "Commands in"=w420, "Mirror"=w390) -> ("error out"=w395:errorcluster)  [unwired: 2 in, 2 out]
                          }
                          frame #4 {
                            n151 = call "DataHaso dtor.vi"("Data Haso"=w436) -> ()  [unwired: 6 in, 1 out]
                          }
                        }
                      }
                      frame #3 {
                        n152 = for {
                          N: "Iteration #" -> [_]
                          tunnel: w452 -> [w481]
                          tunnel: w451 -> [w480]
                          tunnel: w449 -> [w479]
                          tunnel: w448 -> [w478]
                          tunnel: w447 -> [w477]
                          tunnel: [w475] -> w446
                          tunnel: w445 -> [w470]
                          tunnel: [w469] -> w444
                          tunnel: [w467] -> w443
                          tunnel: [w465] -> w442
                          tunnel: [w463] -> w441
                          tunnel: [w460] -> w440
                          tunnel: w439 -> [w459]
                          i -> [w458]
                          n153 = Increment(x=w458) -> (x+1=w457:i32)
                          n154 = flat-sequence {
                            tunnel: [w507] -> w500
                            tunnel: [w508] -> w499
                            tunnel: [w509] -> w498
                            tunnel: [w513] -> w497
                            tunnel: [w512] -> w496
                            tunnel: [w511] -> w495
                            tunnel: [w510] -> w494
                            tunnel: w481 -> [w511]
                            tunnel: w480 -> [w510]
                            tunnel: w479 -> [w509]
                            tunnel: w478 -> [w508]
                            tunnel: w477 -> [w507]
                            tunnel: [w506] -> w471
                            tunnel: w470 -> [w506]
                            tunnel: w457 -> [w504]
                            tunnel: [w503] -> w454
                            tunnel: w500 -> [w540]
                            tunnel: w499 -> [w541]
                            tunnel: w498 -> [w542]
                            tunnel: [w542] -> w493
                            tunnel: [w539] -> w492
                            tunnel: [w538] -> w491
                            tunnel: [w537] -> w490
                            tunnel: w497 -> [w537]
                            tunnel: [w536] -> w489
                            tunnel: w496 -> [w536]
                            tunnel: [w535] -> w488
                            tunnel: w495 -> [w535]
                            tunnel: [w534] -> w487
                            tunnel: w494 -> [w534]
                            tunnel: [w533] -> w472
                            tunnel: w471 -> [w533]
                            tunnel: [w532] -> w455
                            tunnel: w454 -> [w532]
                            tunnel: w493 -> [w555]
                            tunnel: [w555] -> w484
                            tunnel: [w554] -> w485
                            tunnel: w492 -> [w554]
                            tunnel: [w553] -> w486
                            tunnel: w491 -> [w553]
                            tunnel: w490 -> [w548]
                            tunnel: w489 -> [w547]
                            tunnel: [w546] -> w483
                            tunnel: w488 -> [w546]
                            tunnel: [w545] -> w482
                            tunnel: w487 -> [w545]
                            tunnel: [w544] -> w473
                            tunnel: w472 -> [w544]
                            tunnel: [w543] -> w456
                            tunnel: w455 -> [w543]
                            tunnel: w486 -> [w623]
                            tunnel: w485 -> [w624]
                            tunnel: w484 -> [w625]
                            tunnel: w483 -> [w610]
                            tunnel: w482 -> [w609]
                            tunnel: [w589] -> w476
                            tunnel: [w588] -> w474
                            tunnel: w473 -> [w568]
                            tunnel: [w584] -> w468
                            tunnel: [w583] -> w466
                            tunnel: [w582] -> w464
                            tunnel: [w581] -> w462
                            tunnel: [w570] -> w461
                            tunnel: w459 -> [w567]
                            tunnel: w456 -> [w564]
                            tunnel: [w561] -> w453
                            tunnel: w476 -> [w637]
                            tunnel: [w636] -> w475
                            tunnel: w474 -> [w636]
                            tunnel: [w635] -> w469
                            tunnel: w468 -> [w635]
                            tunnel: [w634] -> w467
                            tunnel: w466 -> [w634]
                            tunnel: [w633] -> w465
                            tunnel: w464 -> [w633]
                            tunnel: [w629] -> w463
                            tunnel: w462 -> [w630]
                            tunnel: w461 -> [w632]
                            tunnel: [w632] -> w460
                            tunnel: w453 -> [w631]
                            frame #0 {
                              n155 = local read "Laser Power%(0-100)"() -> (w519:dbl)
                              n156 = local read "AoExp Time"() -> (w518:dbl)
                              n157 = local read "galvo scan?"() -> (w501:bool)
                              n158 = local read "Scale factor"() -> (w502:dbl)
                              n159 = case shown="False" w501 {
                                tunnel: FALSE ("Boolean") -> [w522 w531]
                                tunnel: w519 -> [w524 w530]
                                tunnel: w518 -> [w523 w529]
                                tunnel: [w526 w528] -> w517
                                tunnel: w502 -> [w525 w527]
                                frame False {
                                n160 = call "waveform gen_DC_1.vi"("Scale factor"=w525, "Boolean"=w522, "Exposure Time (s)"=w523, "Laser Power%(0-100)"=w524) -> ("waveform"=w526:waveform(dbl)[])
                                }
                                frame True {
                                n161 = call "waveform gen_scale factor.vi"("Scale factor"=w527, "Boolean"=w531, "Exposure Time (s)"=w529, "Laser Power%(0-100)"=w530) -> ("waveform"=w528:waveform(dbl)[])
                                }
                              }
                              n162 = local read "Iteration #"() -> (w505:u16)
                              n163 = Index Array(array=w517, index=4) -> (element=w516:waveform(dbl))
                              n164 = Less?(x=w505, y=w504) -> (x < y?=w503:bool)
                              n165 = call "AO triggle.vi"("physical channels"=tag "Dev1/ao0:4", "data"=w517, "waveform"=w516, "trig source"=tag "/Dev1/PFI0") -> ("task out"=w513:refnum<k21>, "error out"=w512:errorcluster)  [unwired: 1 in]
                            }
                            frame #1 {
                              n166 = call "Camera Start.vi"("error in (no error)"=w540, "camera"=w541) -> ("error out"=w538:errorcluster, "camera (dup)"=w539:T7)  [unwired: 4 in]
                            }
                            frame #2 {
                              n167 = while {
                                tunnel: [w560] -> w550
                                tunnel: [w559] -> w549
                                tunnel: w548 -> [w557]
                                tunnel: w547 -> [w556]
                                stop <- w558 stop-if-true
                                n168 = call <vilib>:"DAQmx Is Task Done.vi"("task/channels in"=w557, "error in"=w556) -> ("task out"=w560:refnum<k21>, "task done?"=w558:bool, "error out"=w559:errorcluster)  [unwired: 11 in]
                              }
                              n169 = call "DO single value.vi"("data"=TRUE, "lines"=tag "Dev1/port0/line0") -> ()  [unwired: 1 in, 1 out]
                              n170 = call <vilib>:"DAQmx Clear Task.vi"("task in"=w550, "error in"=w549) -> ()  [unwired: 13 in, 1 out]
                            }
                            frame #3 {
                              n171 = call "Camera Get image.vi"("error in (no error)"=w623, "camera"=w624) -> ("error out"=w606:errorcluster, "Image"=w607:T11, "camera (dup)"=w608:T7)  [unwired: 3 in]
                              n172 = call "Camera Stop.vi"("error in (no error)"=w606, "camera"=w608) -> ()  [unwired: 4 in, 2 out]
                              n173 = call "Image get data.vi"("error in (no error)"=w606, "Image Compat"=w607) -> ("error out"=w596:errorcluster, "Array"=w605:u32[][], "Image Compat (dup)"=w595:T11)  [unwired: 3 in]
                              n174 = call "AO single value.vi"("data"=0.0, "physical channels"=tag "Dev1/ao4") -> ()  [unwired: 1 in, 1 out]
                              n175 = local write "Camera image"(w605) -> ()
                              n176 = call "Haso compute slopes.vi"("error in (no error)"=w596, "Image Compat"=w595, "Haso"=w625) -> ("error out"=w573:errorcluster, "Data Haso"=w572:T4)  [unwired: 1 in, 2 out]
                              n177 = call "DO single value.vi"("data"=FALSE, "lines"=tag "Dev1/port0/line0") -> ()  [unwired: 1 in, 1 out]
                              n178 = call "DataHaso get reconstruction prefs.vi"("error in (no error)"=w573, "Data Haso"=w572) -> ("error out"=w579:errorcluster, "Reconstruction Preferences"=w578:T13, "Data Haso (dup)"=w580:T4)  [unwired: 3 in]
                              n179 = Bundle By Name(cluster=w578, "Reconstruction type"=enum16{"Modal", "Zonal"}."Modal", "Polynomial type"=enum16{"Zernike", "Legendre"}."Zernike", "Modal reconstruction prefs.Number of coefficients"=u32 32) -> (w577:T13)
                              n180 = call "DataHaso set reconstruction prefs.vi"("error in (no error)"=w579, "Reconstruction Preferences"=w577, "Data Haso"=w580) -> ("error out"=w565:errorcluster, "Data Haso (dup)"=w566:T4)  [unwired: 3 in]
                              n181 = call "DataHaso get modal coefficients.vi"("error in (no error)"=w565, "Data Haso"=w566) -> ("error out"=w571:errorcluster, "Coefficients (µm)"=w570:sgl[], "Data Haso (dup)"=w569:T4)  [unwired: 3 in]
                              "Model Coefficients (µm) after" <- w570
                              n182 = Bundle By Name(cluster=T3 {"Filtre tilt X"=FALSE, "Filtre tilt Y"=FALSE, "Filtre courbure"=FALSE} ("Filtre"), "Filtre tilt X"="Filter x tilt", "Filtre tilt Y"="Filter y tilt", "Filtre courbure"="Curvature filter") -> (w593:T3)
                              n183 = call "DataHaso parameters.vi"("error in (no error)"=w571, "Data Haso"=w569) -> ("error out"=w603:errorcluster, "Parameters"=w582:T1, "Data Haso (dup)"=w604:T4)  [unwired: 3 in]
                              "after correction" <- w582
                              n184 = control-ref of="after correction"() -> (w587:refnum<vi>)
                              n185 = call "DataHaso filter tilt or curvature.vi"("error in (no error)"=w603, "Filter (default: all true)"=w593, "Data Haso"=w604) -> ("error out"=w601:errorcluster, "Data Haso (dup)"=w602:T4)  [unwired: 3 in]
                              n186 = call "DataHaso phase.vi"("error in (no error)"=w601, "Data Haso"=w602) -> ("error out"=w599:errorcluster, "Phase (µm)"=w600:i32, "Data Haso (dup)"=w586:T4)  [unwired: 3 in]
                              n187 = call "Formatter Intensity Graph.vi"("error in (no error)"=w599, "Intensity Graph"=w587, "Surface with pupil"=w600) -> ("error out"=w597:errorcluster, "Surface with pupil (dup)"=w598:i32)  [unwired: 2 in, 1 out]
                              n188 = call "Surface with pupil get stats.vi"("error in (no error)"=w597, "Surface Avec Pupille"=w598) -> ("error out"=w618:errorcluster, "PV"=w583:sgl, "RMS"=w584:dbl)  [unwired: 2 in, 1 out]
                              "RMS" <- w584
                              "PV" <- w583
                              n189 = Merge Errors(w618, w609) -> (w617:errorcluster)
                              n190 = Bundle By Name(cluster=T6 {"Target for tilt"=0, "Target for focus"=0, "Target for all other aberrations"=0} ("References"), "Target for tilt"=w567, "Target for focus"=w567) -> (w621:T6)
                              n191 = call "DataHaso ctor copie.vi"("error in (no error)"=w617, "DataHaso"=w586) -> ("error out"=w620:errorcluster, "new DataHaso"=w619:T4, "DataHaso (dup)"=w585:T4)  [unwired: 3 in]
                              n192 = call "Casao Compute target.vi"("error in (no error)"=w620, "Targets"=w621, "DataHaso"=w619, "Casao"=w610) -> ("error out"=w615:errorcluster, "DataHaso (dup)"=w589:T4, "Casao (dup)"=w616:T10)  [unwired: 1 out]
                              n193 = Bundle By Name(cluster=T5 {"Measurement"=0, "Target"=0, "Manual target"=0} ("Slopes"), "Measurement"=w585, "Target"=w589) -> (w614:T5)
                              n194 = call "Casao get correction commands.vi"("Casao"=w616, "Slopes"=w614, "error in (no error)"=w615) -> ("Casao (dup)"=w588:T10, "Commands"=w581:sgl[], "error out"=w561:errorcluster)  [unwired: 2 in, 2 out]
                              n195 = case shown="True" w564 {
                                tunnel: w561 -> [_ w628]
                                tunnel: w581 -> [_ w627]
                                tunnel: w568 -> [_ w626]
                                frame False {
                                }
                                frame True {
                                n196 = call "PhaseModul apply command.vi"("error in (no error)"=w628, "Commands in"=w627, "Mirror"=w626) -> ()  [unwired: 2 in, 3 out]
                                }
                              }
                            }
                            frame #4 {
                              n197 = call "DataHaso dtor.vi"("Data Haso"=w637) -> ()  [unwired: 6 in, 1 out]
                              n198 = case shown="Error" w631 {
                                tunnel: w630 -> [w638 _]
                                tunnel: [w638 w639] -> w629
                                frame No Error {
                                }
                                frame Error {
                                n199 = Initialize Array(0.0 ("element"), 52 ("dimension size")) -> (w639:dbl[])
                                }
                              }
                            }
                          }
                        }
                      }
                      frame #4 {
                        n200 = call "DataHaso dtor.vi"("Data Haso"=w647) -> ()  [unwired: 6 in, 1 out]
                        n201 = local read "Slice now"() -> (w652:dbl)
                        n202 = Cluster To Array(cluster=w658) -> (array=w657:sgl[])
                        n203 = Build Array (concatenate)(w659, w660, w657, w649) -> (w665:dbl[])
                        n204 = Number To Decimal String(number=w652) -> (decimal integer string=w662:string)  [unwired: 1 in]
                        n205 = Number To Decimal String(number=w652) -> (decimal integer string=w654:string)  [unwired: 1 in]
                        n206 = call "AO single value.vi"("data"=0.0, "physical channels"=tag "Dev1/ao4") -> ()  [unwired: 1 in, 1 out]
                        n207 = call "AO single value.vi"("data"=-5.0, "physical channels"=tag "Dev1/ao5") -> ()  [unwired: 1 in, 1 out]
                        n208 = local read "output path"() -> (w646:path)
                        n209 = Concatenate Strings("afterC_slice", w662, ".dat") -> (w645:string)
                        n210 = Concatenate Strings("command", w654, ".dat") -> (w643:string)
                        n211 = Build Path(base path=w646, name or relative path=w645) -> (appended path=w644:path)
                        n212 = Build Path(base path=w646, name or relative path=w643) -> (appended path=w642:path)
                        n213 = call-poly <vilib>:"Write To Spreadsheet File.vi"("transpose? (no:F)"=TRUE, "format (%.3f)"="%.6f", "1D data"=w665, "file path (dialog if empty)"=w644) -> ()  [unwired: 4 in, 1 out]
                        n214 = call-poly <vilib>:"Write To Spreadsheet File.vi"("transpose? (no:F)"=TRUE, "format (%.3f)"="%.6f", "1D data"=w648, "file path (dialog if empty)"=w642) -> ()  [unwired: 4 in, 1 out]
                      }
                      frame #5 {
                        n215 = local read "Average Frame #"() -> (w672:dbl)
                        n216 = for {
                          N: w672 -> [_]
                          n217 = local read "stop"() -> (w673:bool)
                          n218 = Not(x=w673) -> (.not. x?=w674:bool)
                          n219 = case shown="True" w674 {
                            frame False {
                            }
                            frame True {
                              n220 = flat-sequence {
                                frame #0 {
                                n221 = local read "Laser Power%(0-100)"() -> (w678:dbl)
                                n222 = local read "galvo scan?"() -> (w676:bool)
                                n223 = local read "ImExp Time (s)"() -> (w679:dbl)
                                n224 = local read "Scale factor"() -> (w677:dbl)
                                n225 = case shown="False" w676 {
                                tunnel: [w696 w700] -> w680
                                tunnel: w679 -> [w693 w699]
                                tunnel: w678 -> [w694 w698]
                                tunnel: w677 -> [w695 w697]
                                tunnel: TRUE ("Boolean") -> [w692 _]
                                frame False {
                                n226 = call "waveform gen_DC_1.vi"("Scale factor"=w695, "Boolean"=w692, "Exposure Time (s)"=w693, "Laser Power%(0-100)"=w694) -> ("waveform"=w696:waveform(dbl)[])
                                }
                                frame True {
                                n227 = call "waveform gen_scale factor.vi"("Scale factor"=w697, "Exposure Time (s)"=w699, "Laser Power%(0-100)"=w698) -> ("waveform"=w700:waveform(dbl)[])  [unwired: 1 in]
                                }
                                }
                                n228 = Index Array(array=w680, index=4) -> (element=w688:waveform(dbl))
                                n229 = call "AO triggle.vi"("physical channels"=tag "Dev1/ao0:4", "data"=w680, "waveform"=w688, "trig source"=tag "/Dev1/PFI0") -> ("task out"=w685:refnum<k21>, "error out"=w682:errorcluster)  [unwired: 1 in]
                                n230 = call "DO single value.vi"("error in"=w682, "data"=TRUE, "lines"=tag "Dev1/port0/line0") -> ("error out"=w681:errorcluster)
                                n231 = while {
                                tunnel: [w705] -> w691
                                tunnel: [w704] -> w690
                                tunnel: w685 -> [w702]
                                tunnel: w681 -> [w701]
                                stop <- w703 stop-if-true
                                n232 = call <vilib>:"DAQmx Is Task Done.vi"("task/channels in"=w702, "error in"=w701) -> ("task out"=w705:refnum<k21>, "task done?"=w703:bool, "error out"=w704:errorcluster)  [unwired: 11 in]
                                }
                                n233 = call <vilib>:"DAQmx Clear Task.vi"("task in"=w691, "error in"=w690) -> ()  [unwired: 13 in, 1 out]
                                }
                                frame #1 {
                                n234 = call "AO single value.vi"("data"=0.0, "physical channels"=tag "Dev1/ao4") -> ()  [unwired: 1 in, 1 out]
                                n235 = call "DO single value.vi"("data"=FALSE, "lines"=tag "Dev1/port0/line0") -> ()  [unwired: 1 in, 1 out]
                                }
                              }
                            }
                          }
                        }
                      }
                      frame #6 {
                        n236 = local read "Step size(um)"() -> (w716:dbl)
                        n237 = Multiply(x=w716, y=10.0) -> (x*y=w714:dbl)
                        n238 = Number To Decimal String(number=w714) -> (decimal integer string=w711:string)  [unwired: 1 in]
                        n239 = Concatenate Strings("movrel z=", w711) -> (w712:string)
                        n240 = call "WriteCmd.vi"("Command"=w712, "VISA resource name"=refnum<visa-resource-name> "COM1") -> ()  [unwired: 1 in, 1 out]
                      }
                      frame #7 {
                        n241 = Wait (ms)(milliseconds to wait=u32 50) -> ()  [unwired: 1 out]
                      }
                    }
                  }
                }
                n242 = call "AO single value.vi"("data"=0.0, "physical channels"=tag "Dev1/ao4") -> ()  [unwired: 1 in, 1 out]
              }
            }
            frame #2 {
              n243 = call "Casao dtor.vi"("Casao"=w718) -> ()  [unwired: 6 in, 1 out]
            }
          }
        }
      }
    }
    frame #2 {
      n244 = local read "Step size(um)"() -> (w726:dbl)
      n245 = local read "Slices #"() -> (w719:dbl)
      n246 = Multiply(x=w726, y=-10.0) -> (x*y=w727:dbl)
      n247 = Multiply(x=w727, y=w719) -> (x*y=w725:dbl)
      n248 = Number To Decimal String(number=w725) -> (decimal integer string=w721:string)  [unwired: 1 in]
      n249 = Concatenate Strings("movrel z=", w721) -> (w722:string)
      n250 = call "AO single value.vi"("data"=0.0, "physical channels"=tag "Dev1/ao4") -> ()  [unwired: 1 in, 1 out]
      n251 = call "WriteCmd.vi"("Command"=w722, "VISA resource name"=refnum<visa-resource-name> "COM1") -> ()  [unwired: 1 in, 1 out]
      n252 = call "DO single value.vi"("data"=FALSE, "lines"=tag "Dev1/port0/line1") -> ()  [unwired: 1 in, 1 out]
      n253 = call "DO single value.vi"("data"=FALSE, "lines"=tag "Dev1/port0/line0") -> ()  [unwired: 1 in, 1 out]
    }
  }
